vi "Post_Joint_States.vi"(4 "node":string) -> ()   [LabVIEW 2013]
doc: "Read all the current joint states (names, positions, velocity, and efforts)"
uses:
  Baxter Examples/Arm Globals.vi
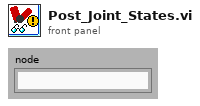
[diagram p1: front panel]
types:
  T1 = typedef "_ROSControl.ctl" = cluster{"topic port":u16, "Node":string, "topic":string, "type":string, "node port":u32, "error ":errorcluster, "Direction":T2, "APIs":string[]}
  T2 = typedef "_ROSDirection.ctl" = enum16{"Node", "Publisher", "Subscriber", "Service Client"}
  T3 = cluster{"Joint Names":string[], "Position":dbl[], "Velocity":dbl[], "Effort":dbl[]}
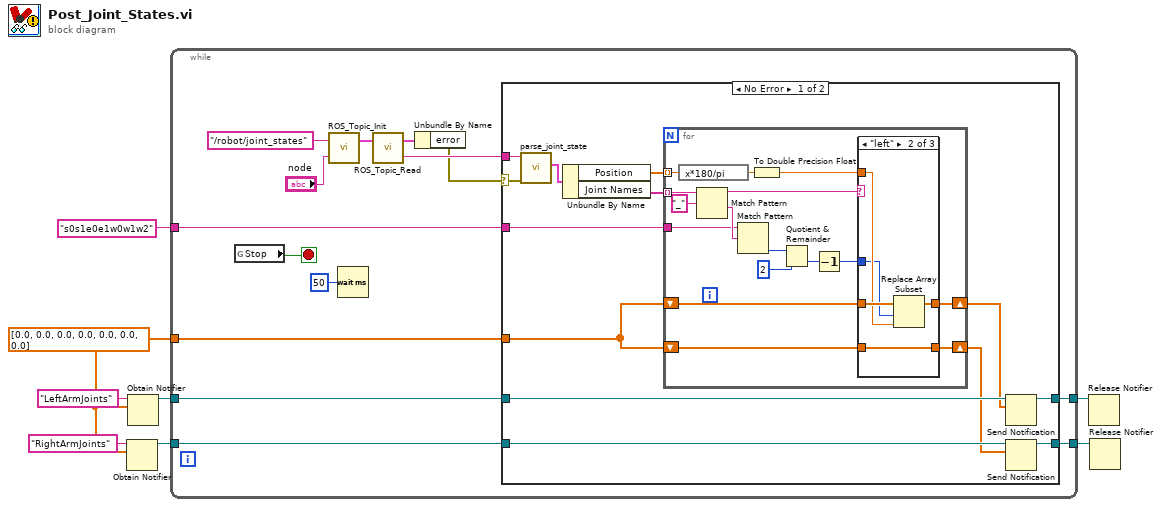
[diagram p0: block diagram]
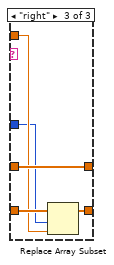
[diagram p3: hidden frame]
diagram:
  w4 = dbl[] [0.0, 0.0, 0.0, 0.0, 0.0, 0.0, 0.0]
  n1 = Obtain Notifier(name (unnamed)="RightArmJoints", notification data type=w4) -> (notifier out=w5:refnum<notifier>)  [unwired: 2 in, 2 out]
  n2 = Obtain Notifier(name (unnamed)="LeftArmJoints", notification data type=w4) -> (notifier out=w6:refnum<notifier>)  [unwired: 2 in, 2 out]
  n3 = while {
    tunnel: w6 -> [w15]
    tunnel: w5 -> [w13]
    tunnel: w4 -> [w17]
    tunnel: [w14] -> w2
    tunnel: [w12] -> w3
    tunnel: "s0s1e0e1w0w1w2" -> [w10]
    stop <- w18 stop-if-true
    n4 = global read "Arm Globals.vi" "Stop"() -> (w18:bool)
    n5 = call "ROS_Topic_Init.vi"("node"="node", "topic"="/robot/joint_states") -> ("ROS out"=w20:T1)  [unwired: 1 in]
    n6 = Wait (ms)(milliseconds to wait=u32 50) -> ()  [unwired: 1 out]
    n7 = call "ROS_Topic_Read.vi"("ROS in"=w20) -> ("Reply"=w11:string, "ROS out"=w19:T1)  [unwired: 1 in]
    n8 = Unbundle By Name(w19) -> ("error"=w9:errorcluster)
    n9 = case shown="No Error" w9 {
      selector: w9 -> [w23 _]
      tunnel: w17 -> [w35 _]
      tunnel: w15 -> [w34 w65]
      tunnel: [w32 w65] -> w14
      tunnel: w13 -> [w31 w64]
      tunnel: [w30 w64] -> w12
      tunnel: w11 -> [w28 _]
      tunnel: w10 -> [w24 _]
      frame No Error {
        n10 = call "parse_joint_state.vi"("error in"=w23, "msg in"=w28) -> ("ROS Joint States"=w27:T3)  [unwired: 2 in, 3 out]
        n11 = Unbundle By Name(w27) -> ("Position"=w26:dbl[], "Joint Names"=w25:string[])
        n12 = for {
          shift-right: [w51] -> w33
          shift-left: w35 -> [w50]
          shift-right: [w48] -> w29
          shift-left: w35 -> [w49]
          tunnel: w25 -> [w44] mode=indexing
          tunnel: w26 -> [w47] mode=indexing
          tunnel: w24 -> [w37]
          n13 = expression code="x*180/pi"(w47) -> (w46:dbl)
          n14 = Match Pattern(string=w44, regular expression="_") -> (before substring=w38:string, after substring=w42:string)  [unwired: 1 in, 2 out]
          n15 = Match Pattern(string=w37, regular expression=w42) -> (offset past match=w41:i32)  [unwired: 1 in, 3 out]
          n16 = To Double Precision Float(number=w46) -> (double precision float=w45:dbl)
          n17 = Quotient & Remainder(x=w41, y=2) -> (floor(x/y)=w39:i32)  [unwired: 1 out]
          n18 = Decrement(x=w39) -> (x-1=w36:i32)
          n19 = case shown="\"left\"" w38 {
            tunnel: [w53 w56 w63] -> w51
            tunnel: w50 -> [w53 w57 w63]
            tunnel: w45 -> [_ w55 w60]
            tunnel: w49 -> [w52 w58 w61]
            tunnel: [w52 w58 w62] -> w48
            tunnel: w36 -> [_ w54 w59]
            frame Default {
            }
            frame "left" {
              n20 = Replace Array Subset(array=w57, new element=w55, index=w54) -> (w56:dbl[])
            }
            frame "right" {
              n21 = Replace Array Subset(array=w61, new element=w60, index=w59) -> (w62:dbl[])
            }
          }
        }
        n22 = Send Notification(notification=w33, notifier=w34) -> (notifier out=w32:refnum<notifier>)  [unwired: 1 in, 1 out]
        n23 = Send Notification(notification=w29, notifier=w31) -> (notifier out=w30:refnum<notifier>)  [unwired: 1 in, 1 out]
      }
      frame Error {
      }
    }
  }
  n24 = Release Notifier(notifier=w2) -> ()  [unwired: 2 in, 3 out]
  n25 = Release Notifier(notifier=w3) -> ()  [unwired: 2 in, 3 out]
